vi "Destroy Event References.vi"(8 "error in (no error)":errorcluster, 11 "Event-References":T1) -> (0 "error out":errorcluster)   [LabVIEW 2018, in "Copy of Actor.lvclass"]
uses:
  Copy of Actor.lvclass
  Event-References.ctl
  Stop.ctl
  Launched.ctl
  Some Request.ctl
  Some Response.ctl
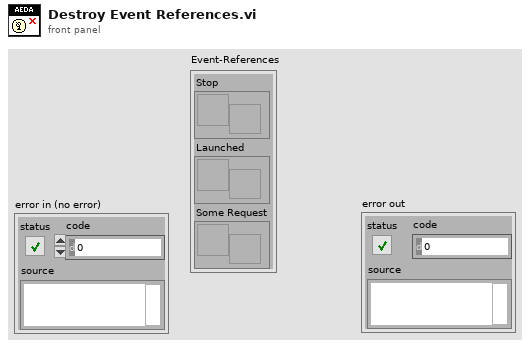
[diagram p1: front panel]
types:
  T1 = typedef "Copy of Actor.lvclass/Event-References.ctl" = cluster{"Stop":refnum<user-event>, "Launched":refnum<user-event>, "Some Request":refnum<user-event>}
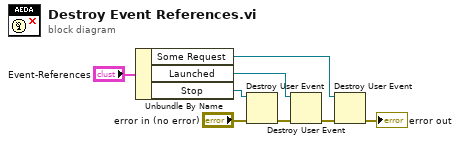
[diagram p0: block diagram]
diagram:
  n1 = Unbundle By Name("Event-References") -> ("Some Request"=w3:refnum<user-event>, "Launched"=w5:refnum<user-event>, "Stop"=w7:refnum<user-event>)
  n2 = Destroy User Event(user event=w7, error in="error in (no error)") -> (error out=w4:errorcluster)
  n3 = Destroy User Event(user event=w5, error in=w4) -> (error out=w2:errorcluster)
  n4 = Destroy User Event(user event=w3, error in=w2) -> (error out=→"error out":errorcluster)
